vi "Format Button Message.vi"(7 "Switch":T1=enum."SW201 - My Cycle") -> (8 "Switch Message":string)   [LabVIEW 2014]
uses:
  type defs/HEUI Switches.ctl
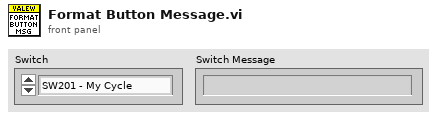
[diagram p1: front panel]
types:
  T1 = typedef "HEUI Switches.ctl" = enum16{"Switch Off /  Reset", "SW201 - My Cycle", "SW202 - Delay Dry", "SW203 - Signal / Volume", "SW204 - Damp Alert", "SW205 - Temp", "SW206 - Ext Tumble", "SW207 - Dryness Level", "SW208 -  (-) Time", "SW209 - Time", "SW210 - (+) Time", "SW211 - eDry ", "SW212 - null", "SW213 - Power", "SW214 - Start / Pause"}
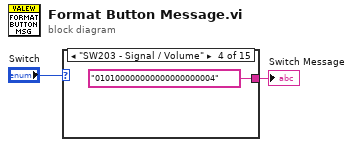
[diagram p0: block diagram]
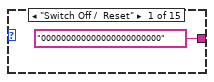
[diagram p2: hidden frame]
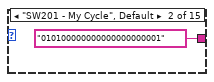
[diagram p3: hidden frame]
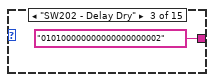
[diagram p4: hidden frame]
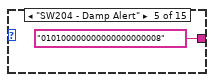
[diagram p5: hidden frame]
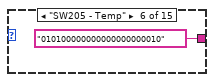
[diagram p6: hidden frame]
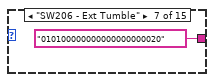
[diagram p7: hidden frame]
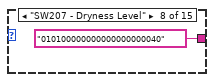
[diagram p8: hidden frame]
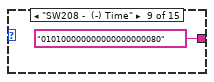
[diagram p9: hidden frame]
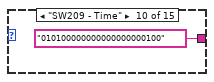
[diagram p10: hidden frame]
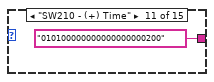
[diagram p11: hidden frame]
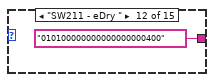
[diagram p12: hidden frame]
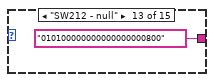
[diagram p13: hidden frame]
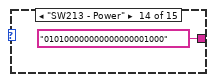
[diagram p14: hidden frame]
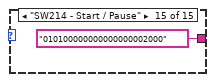
[diagram p15: hidden frame]
diagram:
  n1 = case shown="\"SW203 - Signal / Volume\"" "Switch" {
    tunnel: ["000000000000000000000000" ("Message") "010100000000000000000001" ("Message") "010100000000000000000002" ("Message") "010100000000000000000004" ("Message") "010100000000000000000008" ("Message") "010100000000000000000010" ("Message") "010100000000000000000020" ("Message") "010100000000000000000040" ("Message") "010100000000000000000080" ("Message") "010100000000000000000100" ("Message") "010100000000000000000200" ("Message") "010100000000000000000400" ("Message") "010100000000000000000800" ("Message") "010100000000000000001000" ("Message") "010100000000000000002000" ("Message")] -> w1
    frame "Switch Off /  Reset" {
    }
    frame "SW201 - My Cycle", Default {
    }
    frame "SW202 - Delay Dry" {
    }
    frame "SW203 - Signal / Volume" {
    }
    frame "SW204 - Damp Alert" {
    }
    frame "SW205 - Temp" {
    }
    frame "SW206 - Ext Tumble" {
    }
    frame "SW207 - Dryness Level" {
    }
    frame "SW208 -  (-) Time" {
    }
    frame "SW209 - Time" {
    }
    frame "SW210 - (+) Time" {
    }
    frame "SW211 - eDry " {
    }
    frame "SW212 - null" {
    }
    frame "SW213 - Power" {
    }
    frame "SW214 - Start / Pause" {
    }
  }
  "Switch Message" <- w1
